vi "AE Groups SR Data.vi"(4 "Year":i16, 6 "Week":i16, 8 "error in (no error)":errorcluster, 10 "AE-Groups In":string[](array[string]), 11 "Report DVR in":refnum<data-value>) -> (0 "error out":errorcluster, 1 "Formated SR Data Out":string[][](array[string]), 2 "SRs Out":T1[](array[typedef]) {"Open SRs" scale=0.0..40.0; "Solved in more then 5 Workdays" scale=0.0..40.0; "In Work SRs" scale=0.0..40.0; "Solved Within 5 workdays" scale=0.0..40.0; "New SRs" scale=0.0..40.0}, 3 "Report DVR out":refnum<data-value>)   [LabVIEW 2017, in "DS_Lib.lvlib" / "SRReportParser.lvlib"]
uses:
  SRReportParser.lvlib
  MainFrame/TypeDefs/DisplayCluster.ctl
  Modules/Private Controls/Report Data Cluster.ctl
  Modules/Private Controls/Data Raw.ctl
  Modules/Data Operations.lvlib
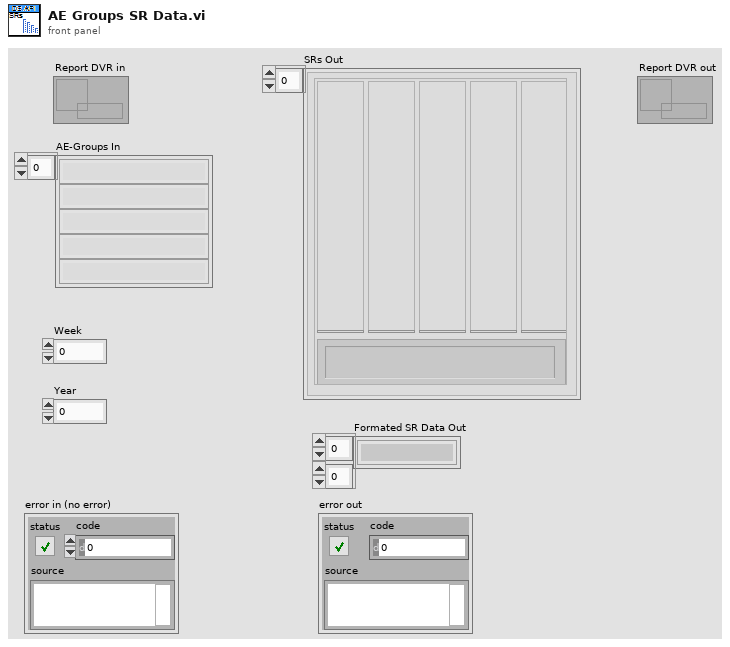
[diagram p1: front panel]
types:
  T1 = typedef "DS_Lib.lvlib/SRReportParser.lvlib/DisplayCluster.ctl" = cluster{"New SRs":u8, "Solved Within 5 workdays":u8, "In Work SRs":u8, "Solved in more then 5 Workdays":u8, "Open SRs":u8, "AE-Team":string}
  T2 = typedef "DS_Lib.lvlib/SRReportParser.lvlib/Weekly_SR_Stats.ctl" = cluster{"AE-Team":string, "In Work SRs":i32, "Open SRs":i32, "Solved within 5 WorkDays":i32, "Solved in more then 5 WorkDays":i32, "New SRs #":i32}
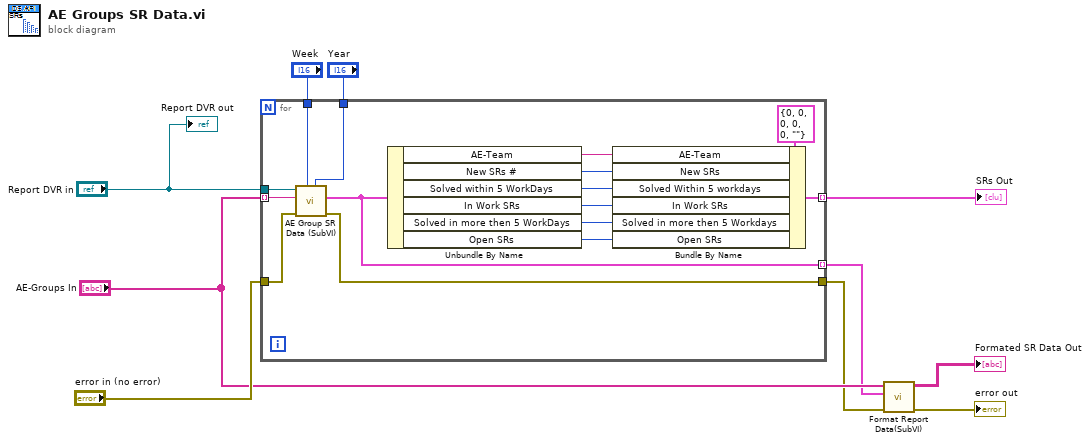
[diagram p0: block diagram]
diagram:
  n1 = for {
    tunnel: "Week" -> [w25]
    tunnel: [w24] -> w7
    tunnel: "AE-Groups In" -> [w23] mode=indexing
    tunnel: "error in (no error)" -> [w22]
    tunnel: [w14] -> w4 mode=indexing
    tunnel: [w13] -> w3 mode=indexing
    tunnel: "Report DVR in" -> [w12]
    tunnel: "Year" -> [w11]
    n2 = call "AE Group SR Data (SubVI).vi"("Year"=w11, "Week"=w25, "error in (no error)"=w22, "AE-Group"=w23, "Report DVR in"=w12) -> ("error out"=w24:errorcluster, "Stats Out"=w13:T2)  [unwired: 5 in]
    n3 = Unbundle By Name(w13) -> ("AE-Team"=w20:string, "New SRs #"=w19:i32, "Solved within 5 WorkDays"=w18:i32, "In Work SRs"=w17:i32, "Solved in more then 5 WorkDays"=w16:i32, "Open SRs"=w15:i32)
    n4 = Bundle By Name(cluster=T1 {"New SRs"=0, "Solved Within 5 workdays"=0, "In Work SRs"=0, "Solved in more then 5 Workdays"=0, "Open SRs"=0, "AE-Team"=""} ("Team"), "AE-Team"=w20, "New SRs"=w19, "Solved Within 5 workdays"=w18, "In Work SRs"=w17, "Solved in more then 5 Workdays"=w16, "Open SRs"=w15) -> (w14:T1)
  }
  "SRs Out" <- w4
  n5 = call "Format Report Data(SubVI).vi"("Error In"=w7, "AE-Groups SR Data"=w3, "AE Group Names"="AE-Groups In") -> ("Error Out"=→"error out":errorcluster, "Formated SR Data Out"=→"Formated SR Data Out":string[][])  [unwired: 5 in, 2 out]
  "Report DVR out" <- "Report DVR in"
